vi "calculate angles.vi"(1 "Midpoint x and y":cluster{"Pos. X":i32, "Pos. Y":i32}, 2 "point":cluster{"Pos. X":i32, "Pos. Y":i32}) -> (0 "angle (degrees)":dbl)   [LabVIEW 2010]
panel:
  out "y":i32
  out "x":i32
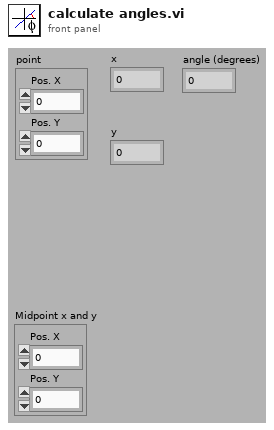
[diagram p1: front panel]
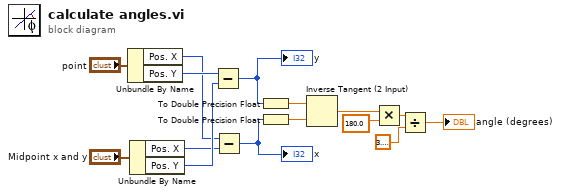
[diagram p0: block diagram]
diagram:
  n1 = Unbundle By Name("point") -> ("Pos. X"=w6:i32, "Pos. Y"=w8:i32)
  n2 = Unbundle By Name("Midpoint x and y") -> ("Pos. X"=w7:i32, "Pos. Y"=w14:i32)
  n3 = Subtract(x=w8, y=w14) -> (x-y=w2:i32)
  "y" <- w2
  n4 = Subtract(x=w6, y=w7) -> (x-y=w1:i32)
  "x" <- w1
  n5 = To Double Precision Float(number=w2) -> (double precision float=w5:dbl)
  n6 = To Double Precision Float(number=w1) -> (double precision float=w4:dbl)
  n7 = Inverse Tangent (2 Input)(1:w4, 2:w5) -> (0:w12:dbl)
  n8 = Multiply(x=w12, y=180.0) -> (x*y=w13:dbl)
  n9 = Divide(x=w13, y=3.141592653589793) -> (x/y=→"angle (degrees)":dbl)
